vi "Get Installed Version.vi"(11 "WebView2 Updater in":refnum<class "WebView2 Updater.lvclass">) -> (0 "error out":errorcluster, 3 "WebView2 Updater out":refnum<class "WebView2 Updater.lvclass">)   [LabVIEW 2020, in "WebView2 Updater.lvclass"]
uses:
  WebView2 Updater.lvclass
  WebView2 Updater.lvclass/WebView2 Updater.ctl
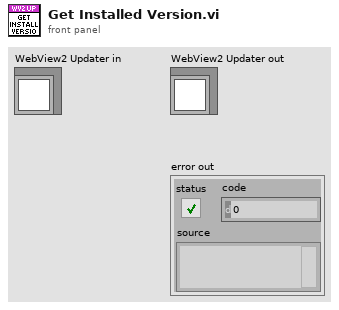
[diagram p1: front panel]
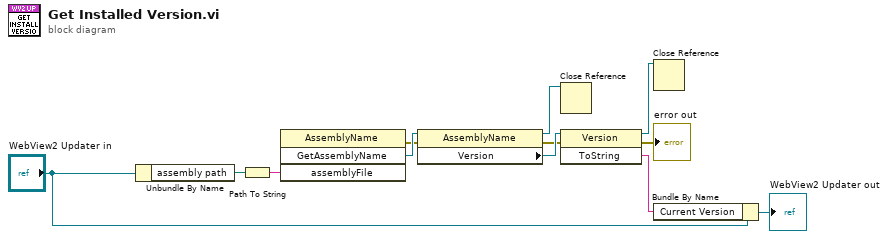
[diagram p0: block diagram]
diagram:
  n1 = Unbundle By Name("WebView2 Updater in") -> ("assembly path"=w2:path)
  n2 = Path To String(path=w2) -> (string=w9:string)
  n3 = invoke class="AssemblyName" method="GetAssemblyName"("assemblyFile"=w9) -> (error out=w6:errorcluster, "GetAssemblyName"=w8:refnum<k24>)  [unwired: 3 in, 2 out]
  n4 = property class="AssemblyName"(reference=w8, error in=w6) -> (reference out=w5:refnum<k24>, error out=w3:errorcluster, "Version"=w7:refnum<k24>)
  n5 = Close Reference(reference=w5) -> ()  [unwired: 1 in, 1 out]
  n6 = invoke class="Version" method="ToString"(reference=w7, error in=w3) -> (reference out=w4:refnum<k24>, error out=→"error out":errorcluster, "ToString"=w11:string)  [unwired: 1 in]
  n7 = Close Reference(reference=w4) -> ()  [unwired: 1 in, 1 out]
  n8 = Bundle By Name(cluster="WebView2 Updater in", "Current Version"=w11) -> (→"WebView2 Updater out":refnum<class "WebView2 Updater.lvclass">)
